vi "Errors.vi"(9 "Error ID":i32, 10 "Done?":bool, 11 "Errors in":bool[](array[boolean])) -> (3 "Erros out":bool[](array[boolean]))   [LabVIEW 2015]
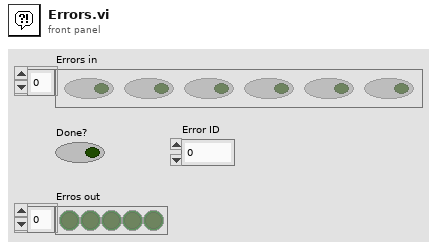
[diagram p1: front panel]
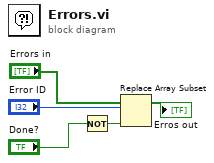
[diagram p0: block diagram]
diagram:
  n1 = Not(x="Done?") -> (.not. x?=w1:bool)
  n2 = Replace Array Subset(array="Errors in", new element=w1, index="Error ID") -> (→"Erros out":bool[])
